vi "UE9 Multiple IO Example Loop.vi"() -> ()   [LabVIEW 2021]
panel:
  out "iterations/sec":dbl format="%.2f"
  out "ms/iteration":dbl format="%.2f"
  in  "stop":bool
  in  "AIN Resolution":i32=12
  in  "FirstFound":bool=TRUE
  in  "ConnectionType":u16(ring) items=["LJ_ctUSB", "LJ_ctETHERNET"]
  in  "Address":string="192.168.1.209"
  out "AIN Readings":dbl[](array[numeric]) format="%.6f"
  out "FIO1":bool
  out "FIO0":bool
  in  "# AIN":i32=8
  in  "Write Values":T1 {"DAC1" format="%.4f"; "DAC0" format="%.4f"}
  out "Error Message":string
  in  "error in":errorcluster
  out "error out":errorcluster
  # "Outputs DAC0-DAC1 and FIO2-FIO3.  Acquires FIO0-FIO1 and specified number of analog inputs\nstarting from AIN0."
  # "Specify an IP address for Ethernet, or Local ID\nfor USB.  If FirstFound is selected, Local ID is\nignored for USB."
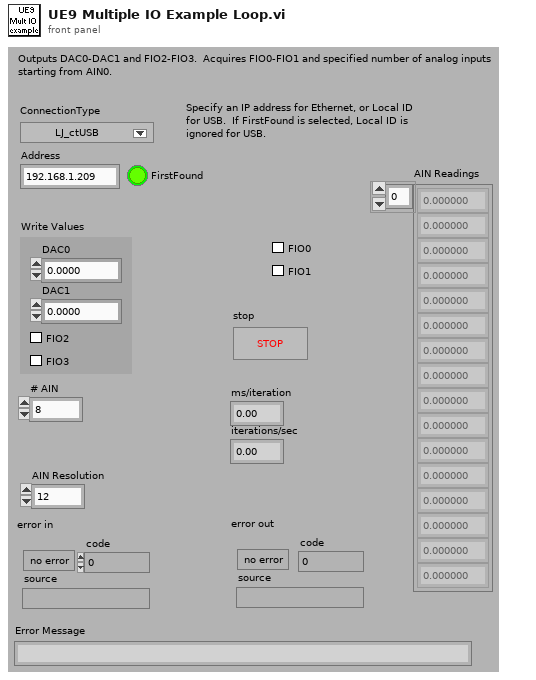
[diagram p1: front panel]
types:
  T1 = cluster{"DAC0":dbl, "DAC1":dbl, "FIO2":bool, "FIO3":bool}
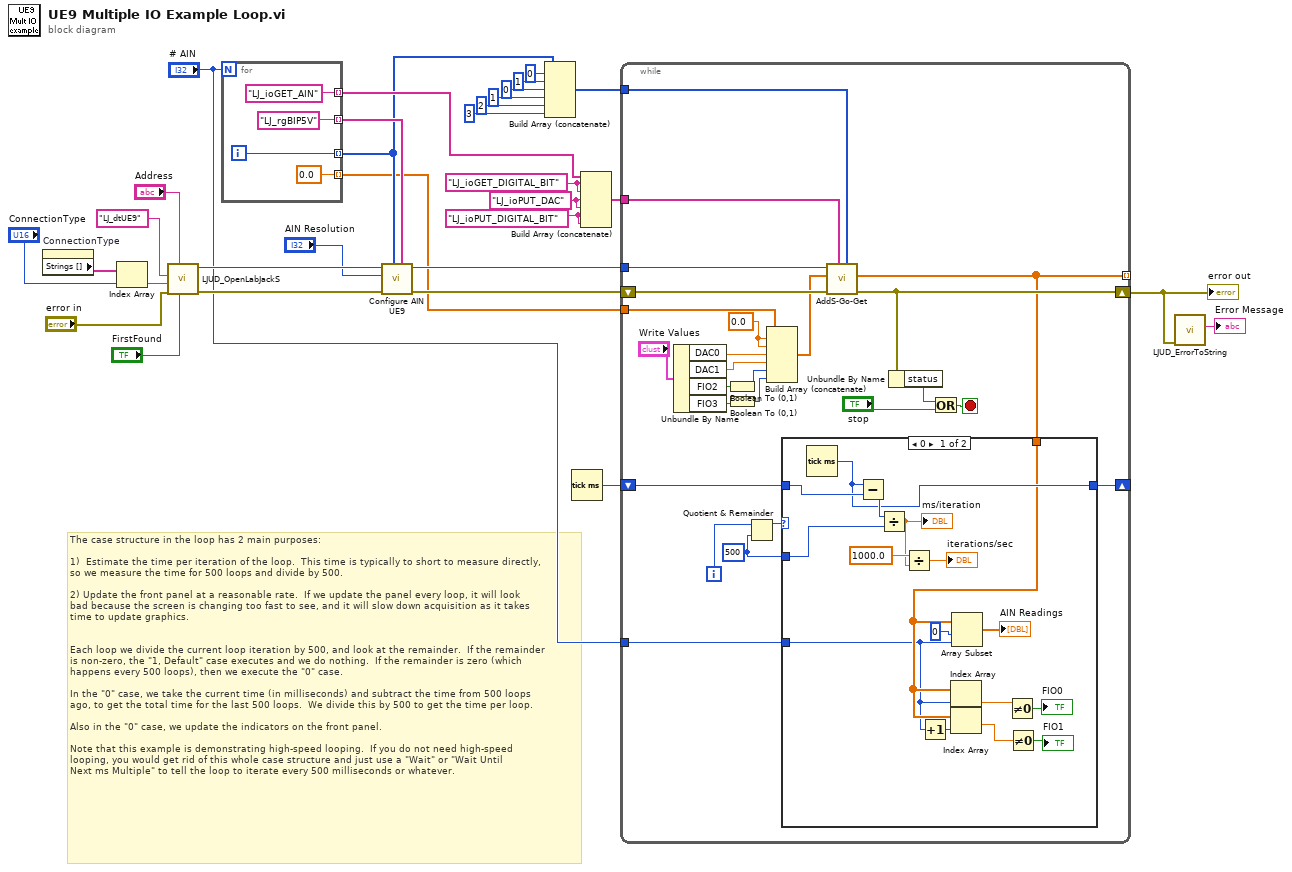
[diagram p0: block diagram]
diagram:
  w26 = "LJ_ioPUT_DIGITAL_BIT" ("IOType")
  w27 = "LJ_ioPUT_DAC" ("IOType")
  w28 = "LJ_ioGET_DIGITAL_BIT" ("IOType")
  # "The case structure in the loop has 2 main purposes:\n\n1)  Estimate the time per iteration of the loop.  This time is typically to short to measure directly,\nso we measure the time for 500 loops and divide by 500.\n\n2) Update the front panel at a reasonable rate.  If we update the panel every loop, it will look\nbad because the screen is changing too fast to see, and it will slow down acquisition as it takes\ntime to update graphics.\n\n\nEach loop we divide the current loop iteration by 500, and look at the remainder.  If the remainder\nis non-zero, the \"1, Default\" case executes and we do nothing.  If the remainder is zero (which\nhappens every 500 loops), then we execute the \"0\" case.\n\nIn the \"0\" case, we take the current time (in milliseconds) and subtract the time from 500 loops\nago, to get the total time for the last 500 loops.  We divide this by 500 to get the time per loop.\n\nAlso in the \"0\" case, we update the indicators on the front panel.\n\nNote that this example is demonstrating high-speed looping.  If you do not need high-speed\nlooping, you would get rid of this whole case structure and just use a \"Wait\" or \"Wait Until\nNext ms Multiple\" to tell the loop to iterate every 500 milliseconds or whatever."
  n1 = property on="ConnectionType" class="Ring (strict)"() -> ("Strings []"=w13:string[])  [unwired: 2 in, 2 out]
  n2 = Index Array(array=w13, index="ConnectionType") -> (element=w11:string)
  n3 = call "LJUD_OpenLabJackS.vi"("FirstFound"="FirstFound", "Address"="Address", "error in"="error in", "ConnectionType"=w11, "DeviceType"="LJ_dtUE9") -> ("error out"=w17:errorcluster, "Handle"=w16:i32)  [unwired: 4 in, 1 out]
  n4 = for {
    N: "# AIN" -> [_]
    tunnel: [w35] -> w6 mode=indexing
    tunnel: ["LJ_rgBIP5V" ("AIN Range")] -> w8 mode=indexing
    tunnel: ["LJ_ioGET_AIN" ("IOType")] -> w7 mode=indexing
    tunnel: [0.0 ("Input Element")] -> w2 mode=indexing
    i -> [w35]
  }
  n5 = call "Configure AIN UE9.vi"("Ranges"=w8, "Channels"=w6, "error in"=w17, "Resolution"="AIN Resolution", "Handle In"=w16) -> ("error out"=w5:errorcluster, "Handle Out"=w29:i32)  [unwired: 5 in]
  n6 = Build Array (concatenate)(w6, 0 ("Input Element"), 1 ("Input Element"), 0 ("Input Element"), 1 ("Input Element"), 2 ("Input Element"), 3 ("Input Element")) -> (w18:i32[])
  n7 = Tick Count (ms)() -> (millisecond timer value=w3:u32)
  n8 = Build Array (concatenate)(w7, w28, w28, w27, w27, w26, w26) -> (w19:string[])
  n9 = while {
    tunnel: "# AIN" -> [w38]
    tunnel: w2 -> [w37]
    shift-left: w3 -> [w48]
    shift-right: [w51] -> _
    shift-left: w5 -> [w53]
    shift-right: [w54] -> w4
    tunnel: [w39] -> _ mode=indexing
    tunnel: w18 -> [w58]
    tunnel: w19 -> [w59]
    tunnel: w29 -> [w60]
    i -> [w52]
    stop <- w57 stop-if-true
    w36 = 0.0 ("Input Element")
    w49 = 500 ("y")
    n10 = Unbundle By Name("Write Values") -> ("DAC0"=w44:dbl, "DAC1"=w45:dbl, "FIO2"=w46:bool, "FIO3"=w47:bool)
    n11 = Boolean To (0,1)(Boolean=w46) -> (0, 1=w41:i16)
    n12 = Boolean To (0,1)(Boolean=w47) -> (0, 1=w42:i16)
    n13 = Quotient & Remainder(x=w52, y=w49) -> (x-y*floor(x/y)=w50:i32)  [unwired: 1 out]
    n14 = Build Array (concatenate)(w37, w36, w36, w44, w45, w41, w42) -> (w40:dbl[])
    n15 = call "AddS-Go-Get.vi"("Channels"=w58, "IOTypes"=w59, "error in"=w53, "Values Write"=w40, "Handle In"=w60) -> ("error out"=w54:errorcluster, "Values Read"=w39:dbl[])  [unwired: 4 in, 1 out]
    n16 = case shown="0" w50 {
      tunnel: [w70 w77] -> w51
      tunnel: w49 -> [w75 _]
      tunnel: w48 -> [w71 w77]
      tunnel: w39 -> [w62 _]
      tunnel: w38 -> [w61 _]
      frame 0 {
        n17 = Tick Count (ms)() -> (millisecond timer value=w70:u32)
        n18 = Subtract(x=w70, y=w71) -> (x-y=w76:u32)
        n19 = Divide(x=w76, y=w75) -> (x/y=w73:dbl)
        "ms/iteration" <- w73
        n20 = Divide(x=1000.0, y=w73) -> (x/y=→"iterations/sec":dbl)
        n21 = Increment(x=w61) -> (x+1=w65:i32)
        n22 = Index Array(array=w62, index=w61) -> (element=w63:dbl)
        n23 = Index Array(array=w62, index=w65) -> (element=w64:dbl)
        n24 = Array Subset(array=w62, index=0 ("Array Index"), length=w61) -> (→"AIN Readings":dbl[])
        n25 = Not Equal To 0?(x=w63) -> (x != 0?=→"FIO0":bool)
        n26 = Not Equal To 0?(x=w64) -> (x != 0?=→"FIO1":bool)
      }
      frame 1, Default {
      }
    }
    n27 = Unbundle By Name(w54) -> ("status"=w55:bool)
    n28 = Or(x=w55, y="stop") -> (x .or. y?=w57:bool)
  }
  "error out" <- w4
  n29 = call "LJUD_ErrorToString.vi"("error in"=w4) -> ("String"=→"Error Message":string)  [unwired: 10 in]
